vi "CaptPT02-03.vi"(6 "Graph in 2":cluster{dbl[], dbl[]}, 7 "Index":i32=250, 8 "error in":errorcluster, 9 "Length 2":i32=250, 11 "ON 2":bool) -> (0 "error out":errorcluster, 2 "Values 2":cluster{dbl[], dbl[]})   [LabVIEW 2012]
uses:
  GlobalVariables/PT02Parameters.vi
  GlobalVariables/PT03Parameters.vi
  GlobalVariables/CommunicationActivity.vi
  GlobalVariables/ZeroTimeGraph.vi
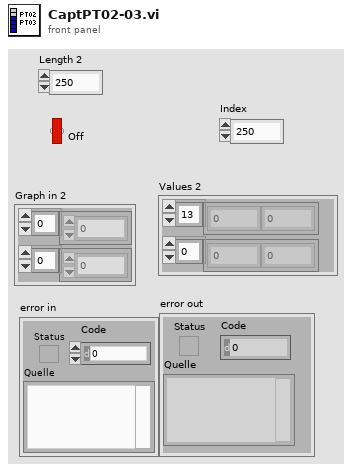
[diagram p1: front panel]
types:
  T1 = cluster{"baudrate":u32, "Port":string, "Timeout":u32, "PressureLimit":dbl, "Slave Address":u8}
  T2 = cluster{"KellerActive":bool, "GantnerActive":bool, "BrooksActive":bool}
  T3 = cluster{bool, "GantnerActive":bool, "BrooksActive":bool}
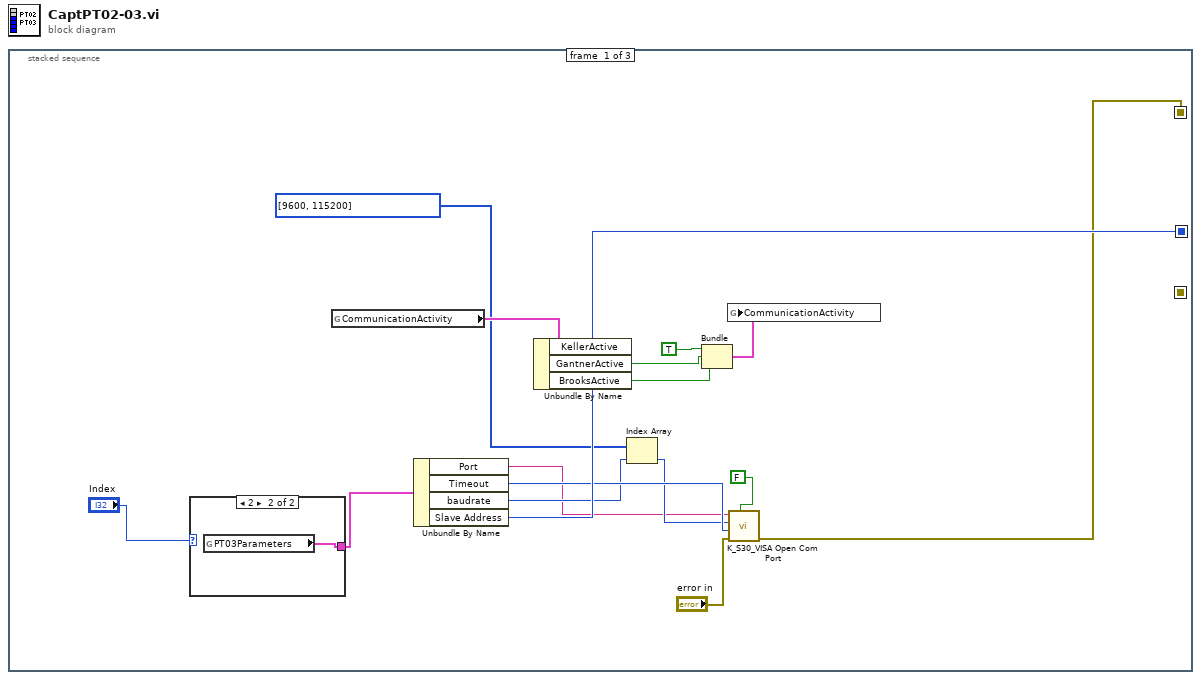
[diagram p0: block diagram]
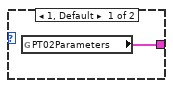
[diagram p2: hidden frame]
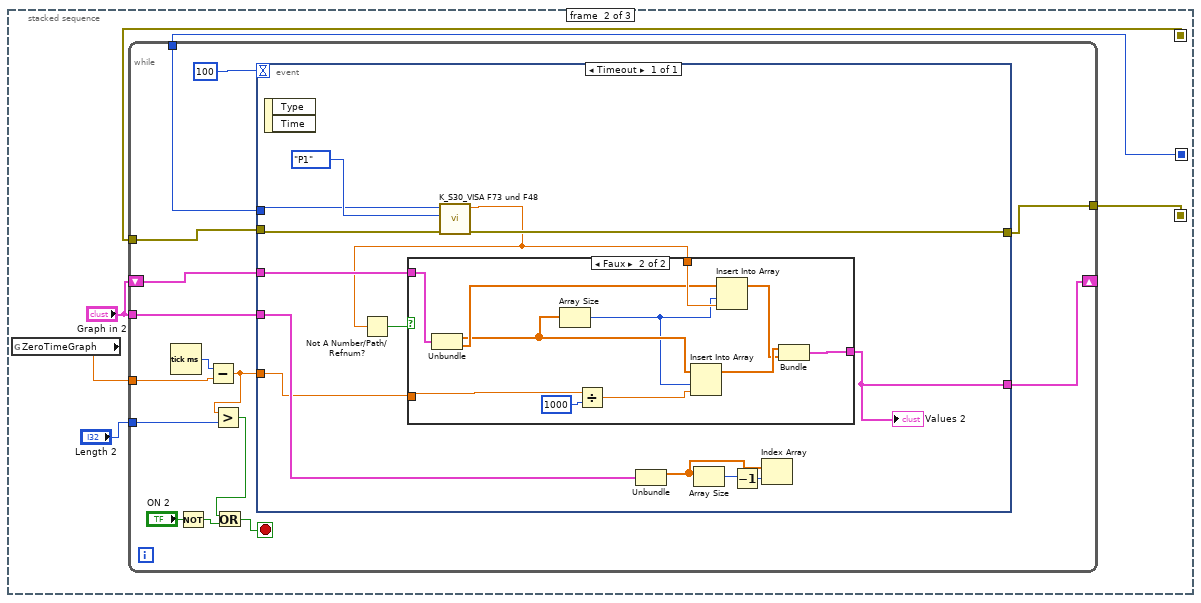
[diagram p3: hidden frame]
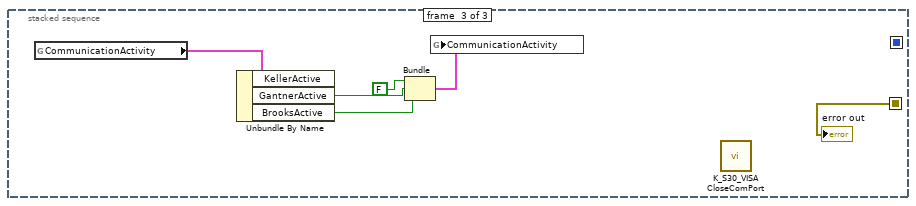
[diagram p5: hidden frame]
diagram:
  n1 = stacked-sequence {
    seq-local: [w8 _ _] -> [_ w20 _]
    seq-local: [_ w21 _] -> [_ _ w70]
    seq-local: [w9 _ _] -> [_ w24 _]
    frame #0 {
      n2 = case shown="2" "Index" {
        tunnel: [w17 w18] -> w14
        frame 1, Default {
          n3 = global read "PT02Parameters.vi" "PT02Parameters"() -> (w17:T1)
        }
        frame 2 {
          n4 = global read "PT03Parameters.vi" "PT03Parameters"() -> (w18:T1)
        }
      }
      n5 = global read "CommunicationActivity.vi" "CommunicationActivity"() -> (w16:T2)
      n6 = Unbundle By Name(w14) -> ("Port"=w1:string, "Timeout"=w5:u32, "baudrate"=w3:u32, "Slave Address"=w9:u8)
      n7 = Unbundle By Name(w16) -> ("GantnerActive"=w11:bool, "BrooksActive"=w12:bool)  [unwired: 1 out]
      n8 = Index Array(array=i32[] [9600, 115200], index=w3) -> (element=w2:i32)
      n9 = Bundle(TRUE, "GantnerActive"=w11, "BrooksActive"=w12) -> (w15:T3)  [unwired: 1 in]
      n10 = global write "CommunicationActivity.vi" "CommunicationActivity"(w15) -> ()
      n11 = call "K_S30_VISA Open Com Port.vi"("RS-converter:\necho"=FALSE ("RS-converter: echo"), "error in (no error)"="error in", "timeout"=w5, "Baudrate"=w2, "VISA resource name"=w1) -> ("error out"=w8:errorcluster)  [unwired: 3 in, 1 out]
    }
    frame #1 {
      n12 = global read "ZeroTimeGraph.vi" "ZeroTimeGraph"() -> (w19:dbl)
      n13 = while {
        tunnel: w20 -> [w38]
        tunnel: w24 -> [w37]
        shift-right: [w33] -> _
        shift-left: "Graph in 2" -> [w36]
        tunnel: "Graph in 2" -> [w35]
        tunnel: "Length 2" -> [w30]
        tunnel: [w26] -> w21
        tunnel: w19 -> [w25]
        stop <- w27 stop-if-true
        n14 = Tick Count (ms)() -> (millisecond timer value=w34:u32)
        n15 = Not(x="ON 2") -> (.not. x?=w31:bool)
        n16 = Subtract(x=w34, y=w25) -> (x-y=w29:dbl)
        n17 = Greater?(x=w29, y=w30) -> (0:w28:bool)
        n18 = Or(x=w28, y=w31) -> (x .or. y?=w27:bool)
        n19 = event shown="[0] Timeout" {
          selector: _ -> [_]
          dyn-events: _ -> [_]
          timeout: 100 -> [_]
          tunnel: w38 -> [w51]
          tunnel: w37 -> [w50]
          tunnel: [w49] -> w26
          tunnel: w36 -> [w44]
          tunnel: w35 -> [w43]
          tunnel: w29 -> [w42]
          tunnel: [w40] -> w33
          event Timeout {
            n20 = event-data() -> ()  [unwired: 1 in, 2 out]
            n21 = call "K_S30_VISA F73 und F48.vi"("error in"=w51, "Channel"=enum16{"CH0", "P1", "P2", "T", "TOB1", "TOB2"}."P1" ("Channel 2"), "Address"=w50) -> ("error out"=w49:errorcluster, "Value"=w41:sgl)  [unwired: 1 in, 2 out]
            n22 = Not A Number/Path/Refnum?(number/path/refnum=w41) -> (NaN/Path/Refnum?=w45:bool)
            n23 = case shown="Faux" w45 {
              tunnel: w42 -> [_ w64]
              tunnel: w41 -> [_ w62]
              tunnel: w44 -> [w53 w61]
              tunnel: [w53 w60] -> w40
              frame True {
              }
              frame False {
                n24 = Unbundle(w61) -> (w56:dbl[], w57:dbl[])
                n25 = Array Size(array=w56) -> (size(s)=w55:i32)
                n26 = Divide(x=w64, y=1000) -> (x/y=w54:dbl)
                n27 = Insert Into Array(array=w56, index=w55, new element=w54) -> (w59:dbl[])
                n28 = Insert Into Array(array=w57, index=w55, new element=w62) -> (w58:dbl[])
                n29 = Bundle(w59, w58) -> (w60:cluster{dbl[], dbl[]})  [unwired: 1 in]
              }
            }
            "Values 2" <- w40
            n30 = Unbundle(w43) -> (w46:dbl[])  [unwired: 1 out]
            n31 = Array Size(array=w46) -> (size(s)=w48:i32)
            n32 = Decrement(x=w48) -> (x-1=w47:i32)
            n33 = Index Array(array=w46, index=w47) -> ()  [unwired: 1 out]
          }
        }
      }
    }
    frame #2 {
      n34 = global read "CommunicationActivity.vi" "CommunicationActivity"() -> (w69:T2)
      n35 = Unbundle By Name(w69) -> ("GantnerActive"=w65:bool, "BrooksActive"=w66:bool)  [unwired: 1 out]
      n36 = Bundle(FALSE, "GantnerActive"=w65, "BrooksActive"=w66) -> (w68:T3)  [unwired: 1 in]
      n37 = global write "CommunicationActivity.vi" "CommunicationActivity"(w68) -> ()
      n38 = call "K_S30_VISA CloseComPort.vi"() -> ()  [unwired: 7 in, 1 out]
      "error out" <- w70
    }
  }
